vi "updateActuator.vi"(8 "error in (no error)":errorcluster, 11 "Model in":refnum<class "Model.lvclass">) -> (0 "error out":errorcluster, 3 "Model out":refnum<class "Model.lvclass">)   [LabVIEW 2015, in "Model.lvclass"]
uses:
  Model.lvclass
  ActuatorCylinder/PressureServoActuatorCylinder/PressureServoCylinderActuator.lvclass
  Model.lvclass/Model.ctl
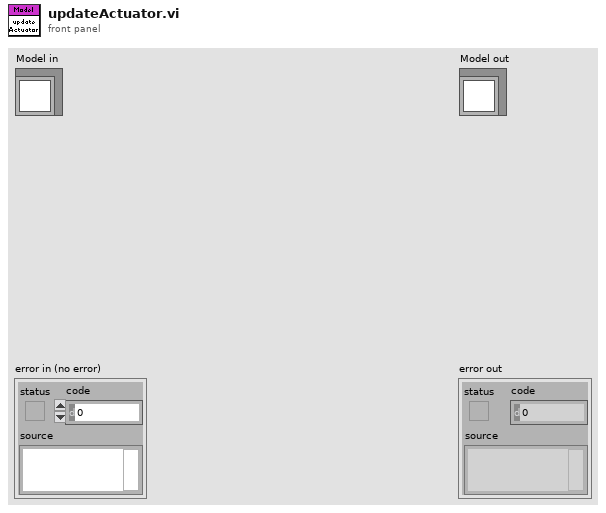
[diagram p1: front panel]
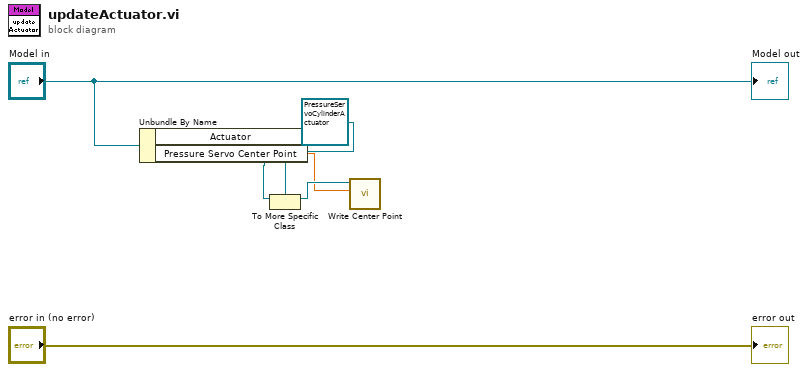
[diagram p0: block diagram]
diagram:
  n1 = Unbundle By Name("Model in") -> ("Actuator"=w4:refnum<class "IActuator.lvclass">, "Pressure Servo Center Point"=w1:dbl[unit])
  n2 = To More Specific Class(target class=refnum<class "PressureServoCylinderActuator.lvclass"> refnum ("PressureServoCylinderActuator.lvclass"), reference=w4) -> (specific class reference=w3:refnum<class "PressureServoCylinderActuator.lvclass">)  [unwired: 1 in, 1 out]
  n3 = call "Write Center Point.vi"("Center Point"=w1, "PressureServoCylinderActuator in"=w3) -> ()  [unwired: 9 in, 1 out]
  "error out" <- "error in (no error)"
  "Model out" <- "Model in"
